vi "Add Connection To Connection List.vi"(8 "error in (no error)":errorcluster, 10 "data value reference":refnum<data-value>, 11 "TCP slave in":refnum<class "TCP Slave.lvclass">) -> (0 "error out":errorcluster)   [LabVIEW 2020, in "SubVIs.lvlib" / "TCP Slave.lvclass"]
uses:
  <vilib>/Modbus/subvis/Protocol/TCP/TCP Slave/TCP Slave.lvclass
  <vilib>/Modbus/subvis/Protocol/TCP/TCP Slave/TCP Slave.lvclass/TCP Slave.ctl
  <vilib>/Modbus/subvis/Protocol/TCP/TCP Slave/Remove Connection Record Reference.vi
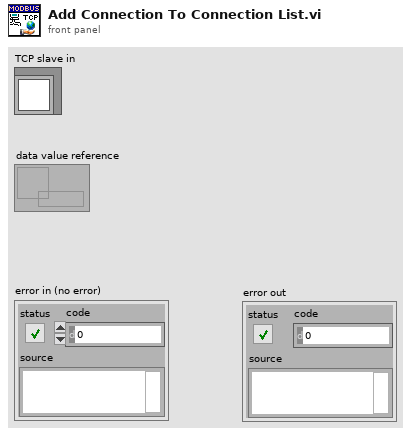
[diagram p1: front panel]
types:
  T1 = typedef "SubVIs.lvlib/TCP Slave.lvclass/Connection Counter.ctl" = cluster{"Currently Connected":u32, "Connection Records":refnum<data-value>[]}
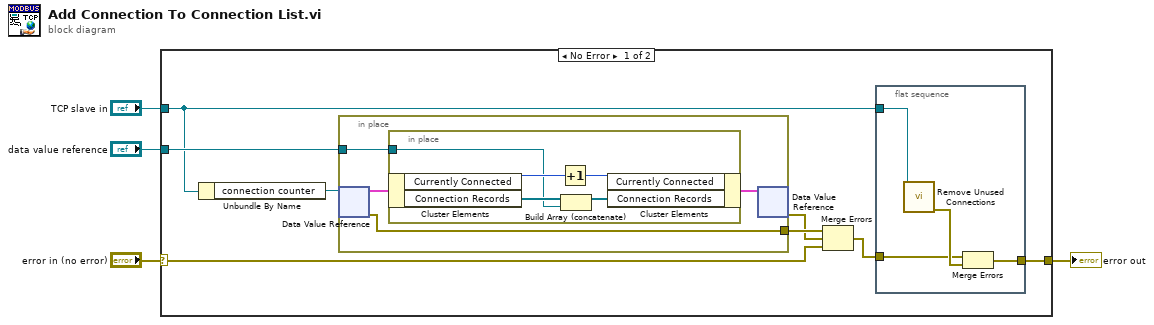
[diagram p0: block diagram]
diagram:
  n1 = case shown="No Error" "error in (no error)" {
    selector: "error in (no error)" -> [w8 w26]
    tunnel: "data value reference" -> [w12 _]
    tunnel: [w5 w26] -> w1
    tunnel: "TCP slave in" -> [w6 _]
    frame No Error {
      n2 = Unbundle By Name(w6) -> ("connection counter"=w11:refnum<data-value>)
      n3 = in-place {
        in-place-border: w12 -> [w18]
        in-place-border: [w17] -> w10
        n4 = in-place-dvr #1(w11) -> (w20:T1, w17:errorcluster)
        n5 = in-place {
          in-place-border: w18 -> [w21]
          n6 = in-place-cluster #2(w20) -> ("Currently Connected"=w25:u32, "Connection Records"=w23:refnum<data-value>[])
          n7 = Increment(x=w25) -> (x+1=w24:u32)
          n8 = Build Array (concatenate)(w23, w21) -> (w22:refnum<data-value>[])
          n9 = in-place-cluster #2("Currently Connected"=w24, "Connection Records"=w22) -> (w19:T1)
        }
        n10 = in-place-dvr #1(w19) -> (w9:errorcluster)  [unwired: 1 out]
      }
      n11 = Merge Errors(w10, w9, w8) -> (w7:errorcluster)
      n12 = flat-sequence {
        tunnel: [w16] -> w5
        tunnel: w7 -> [w14]
        tunnel: w6 -> [w13]
        frame #0 {
          n13 = call <vilib>:"Remove Unused Connections.vi"("TCP slave in"=w13) -> ("error out"=w15:errorcluster)  [unwired: 10 in]
          n14 = Merge Errors(w14, w15) -> (w16:errorcluster)
        }
      }
    }
    frame Error {
    }
  }
  "error out" <- w1
